vi "Servo_serial_mac.vi"() -> ()   [LabVIEW 2017]
uses:
  <vilib>/Instr/_visa.llb/VISA Configure Serial Port (Instr).vi
panel:
  in  "Baud Rate":i32(ring) items=["2400"=2400, "4800"=4800, "9600"=9600, "14400"=14400, "19200"=19200, "28800"=28800, "38400"=38400, "57600"=57600, "115200"=115200]
  in  "Delay (ms)":dbl
  in  "Servo 5":dbl(knob) scale=0.0..180.0
  in  "Servo 4":dbl(knob) scale=0.0..180.0
  in  "Servo 3":dbl(knob) scale=0.0..180.0
  in  "Servo 2":dbl(knob) scale=0.0..180.0
  in  "Servo 1":dbl(knob) scale=0.0..180.0
  in  "Stop":bool
  out "Servo string sent to Arduino":string
  in  "COM Port":refnum<visa-resource-name>
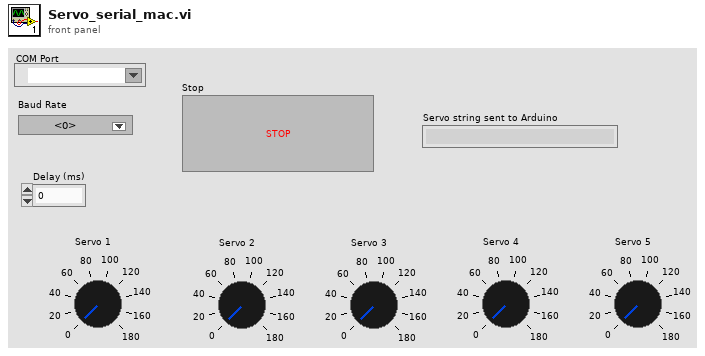
[diagram p1: front panel]
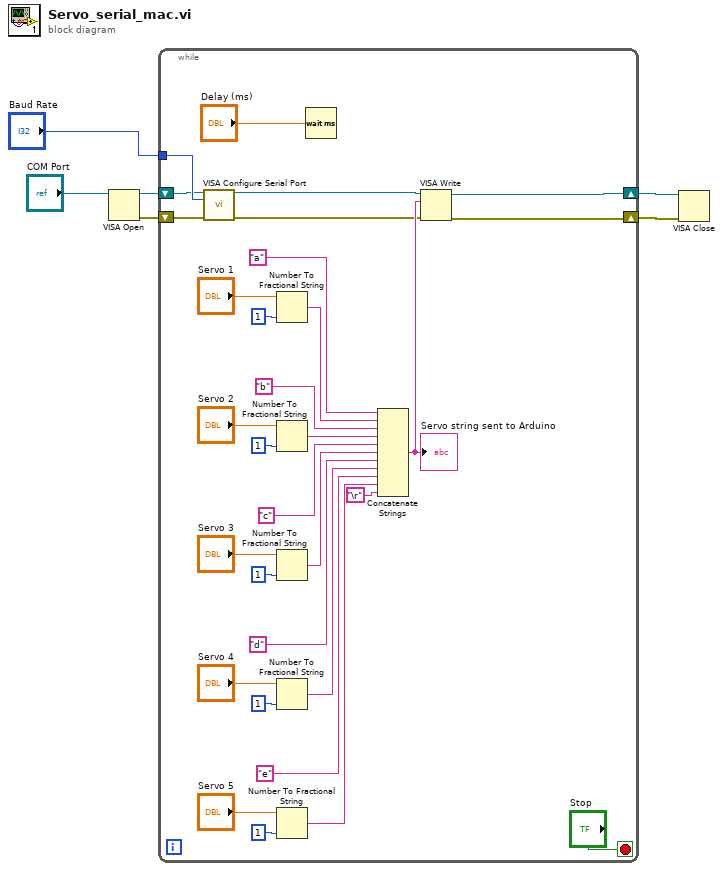
[diagram p0: block diagram]
diagram:
  n1 = VISA Open(VISA resource name="COM Port") -> (VISA resource name=w5:refnum<visa-resource-name>, error out=w4:errorcluster)  [unwired: 4 in]
  n2 = while {
    tunnel: "Baud Rate" -> [w36]
    shift-right: [w14] -> w3
    shift-left: w5 -> [w34]
    shift-right: [w15] -> w2
    shift-left: w4 -> [w33]
    stop <- "Stop" stop-if-true
    n3 = call-poly "VISA Configure Serial Port"("VISA resource name"=w34, "baud rate (9600)"=w36, "error in (no error)"=w33) -> ("VISA resource name out"=w16:refnum<visa-resource-name>, "error out"=w11:errorcluster)  [unwired: 11 in]
    n4 = Number To Fractional String(number="Servo 1", precision (6)=1) -> (F-format string=w32:string)  [unwired: 2 in]
    n5 = Number To Fractional String(number="Servo 2", precision (6)=1) -> (F-format string=w30:string)  [unwired: 2 in]
    n6 = Number To Fractional String(number="Servo 3", precision (6)=1) -> (F-format string=w28:string)  [unwired: 2 in]
    n7 = Number To Fractional String(number="Servo 4", precision (6)=1) -> (F-format string=w18:string)  [unwired: 2 in]
    n8 = Number To Fractional String(number="Servo 5", precision (6)=1) -> (F-format string=w17:string)  [unwired: 2 in]
    n9 = Wait (ms)(milliseconds to wait="Delay (ms)") -> ()  [unwired: 1 out]
    n10 = Concatenate Strings("a", w32, "b", w30, "c", w28, "d", w18, "e", w17, "\r") -> (w37:string)
    "Servo string sent to Arduino" <- w37
    n11 = VISA Write(VISA resource name=w16, write buffer=w37, error in (no error)=w11) -> (VISA resource name out=w14:refnum<visa-resource-name>, error out=w15:errorcluster)  [unwired: 1 out]
  }
  n12 = VISA Close(VISA resource name=w3, error in (no error)=w2) -> ()  [unwired: 1 out]
